vi "BRig_dataRT_stats__T2R_cur.vi"() -> (2 "output_T2R_cur":i32)   [LabVIEW 2014]
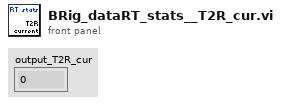
[diagram p1: front panel]
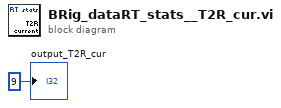
[diagram p0: block diagram]
diagram:
  "output_T2R_cur" <- 9 ("output_iBlock")
